vi "Complex To Cartesian - CM.vi"(0 "Complex Matrix R + Ii":T2) -> (1 "Real Matrix R":T1, 2 "Real Matrix I":T1)   [LabVIEW 2014, in "NI_Matrix.lvlib"]
doc: "Breaks a complex number into its rectangular components."
uses:
  NI_Matrix.lvlib
  ComplexMatrix.ctl
  RealMatrix.ctl
  Array To Matrix - RA2.vi
  Matrix To Array - CM.vi
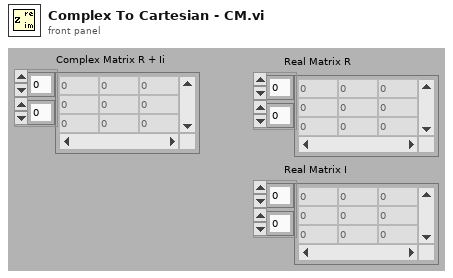
[diagram p1: front panel]
types:
  T1 = typedef "NI_Matrix.lvlib/RealMatrix.ctl" = dbl[][]
  T2 = typedef "NI_Matrix.lvlib/ComplexMatrix.ctl" = cdb[][]
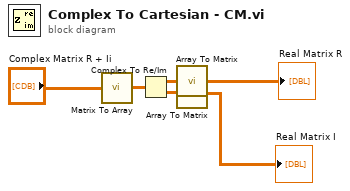
[diagram p0: block diagram]
diagram:
  n1 = call-poly "Matrix To Array.vi"("Complex Matrix"="Complex Matrix R + Ii") -> ("Complex 2D Array"=w6:cdb[][])
  n2 = Complex To Re/Im(x + iy=w6) -> (x=w4:dbl[][], y=w2:dbl[][])
  n3 = call-poly "Array To Matrix.vi"("Real 2D Array"=w4) -> ("Real Matrix"=→"Real Matrix R":T1)
  n4 = call-poly "Array To Matrix.vi"("Real 2D Array"=w2) -> ("Real Matrix"=→"Real Matrix I":T1)
